vi "Read Virtual Memory.vi"(8 "error in (no error)":errorcluster, 11 "1553 Component in":refnum<class "1553 Component.lvclass">) -> (0 "error out":errorcluster, 2 "Virtual Memory Unit":refnum<class "Virtual Memory Unit.lvclass">, 3 "1553 Component out":refnum<class "1553 Component.lvclass">)   [LabVIEW 2020, in "BCI-1553 API.lvlib" / "1553 Component.lvclass"]
doc: "Returns the Virtual Memory that is being used by this component. Virtual Memory is a 1:1 local representation of the data that will eventually be written to the 1553 Session hardware."
uses:
  1553 Component.lvclass
  Dependencies/Virtual Memory Unit/Virtual Memory Unit.lvclass
  1553 Component.lvclass/1553 Component.ctl
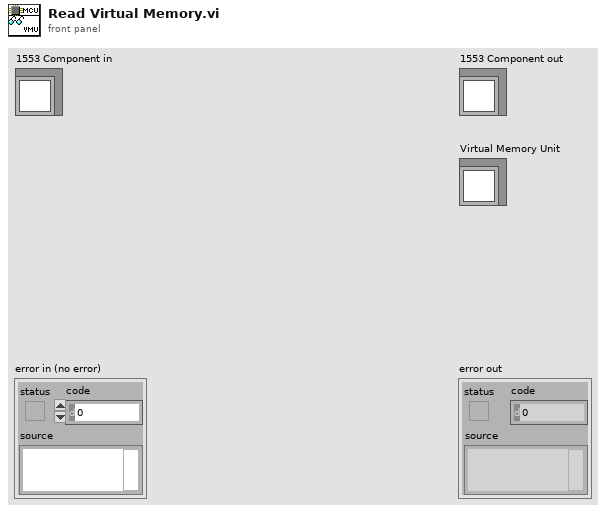
[diagram p1: front panel]
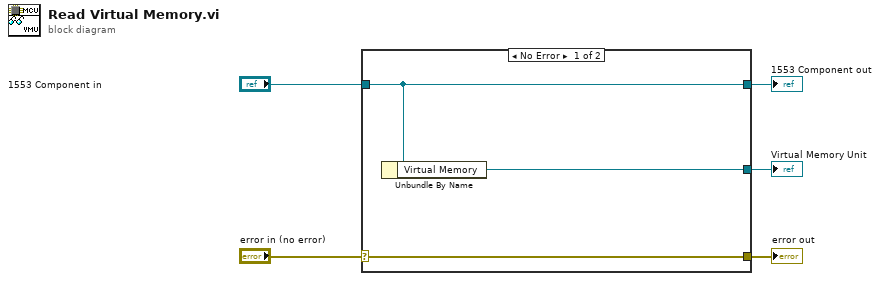
[diagram p0: block diagram]
diagram:
  n1 = case shown="No Error" "error in (no error)" {
    selector: "error in (no error)" -> [w8 w9]
    tunnel: [w8 w9] -> w4
    tunnel: [w7 w10] -> w2
    tunnel: "1553 Component in" -> [w7 w10]
    tunnel: [w6 _] -> w1
    frame No Error {
      n2 = Unbundle By Name(w7) -> ("Virtual Memory"=w6:refnum<class "Virtual Memory Unit.lvclass">)
    }
    frame Error {
    }
  }
  "error out" <- w4
  "1553 Component out" <- w2
  "Virtual Memory Unit" <- w1
